vi "getSubscriberlistfromcluster.vi"(2 "add variables to subscribe":string, 3 "Data cluster out":T1) -> (0 "remote subscriber string":string, 1 "final subscriber string":string)   [LabVIEW 2013]
uses:
  dataCluster.ctl
  <vilib>/vision/Image Controls.llb/IMAQ Image.ctl
  DataQueueTypeDef.ctl
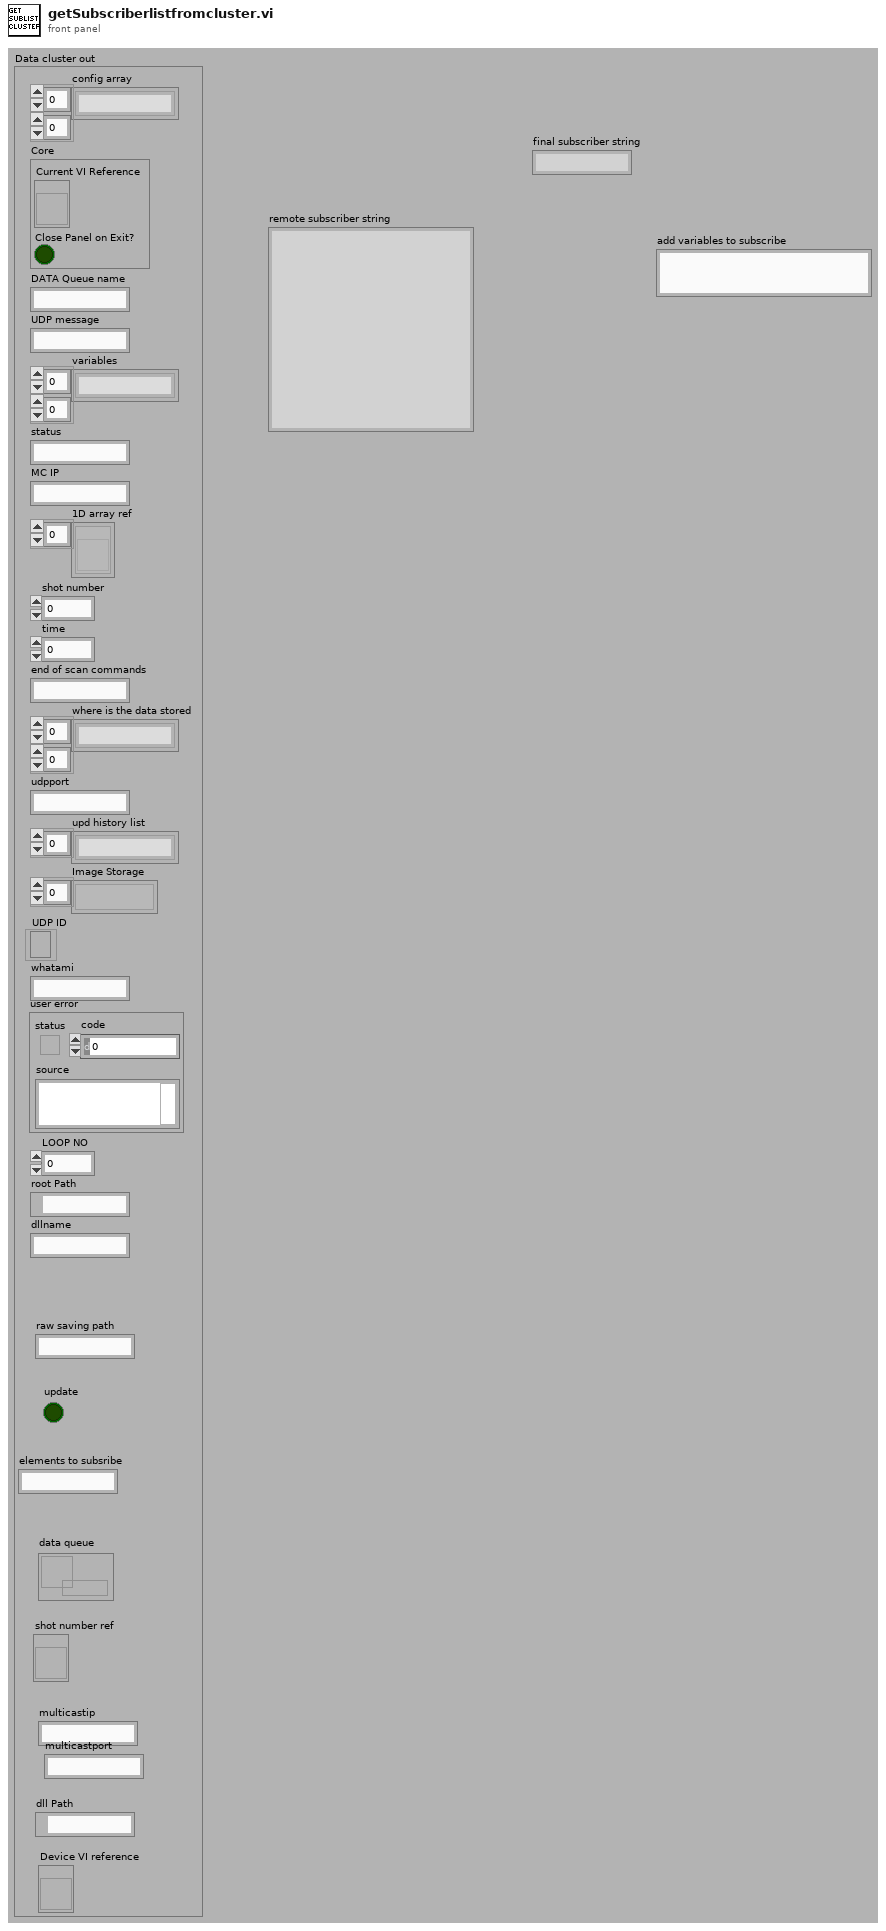
[diagram p1: front panel]
types:
  T1 = typedef "dataCluster.ctl" = cluster{"config array":string[][], "Core":cluster{"Current VI Reference":refnum<vi>, "Close Panel on Exit?":bool}, "DATA Queue name":string, "UDP message":string, "variables":string[][], "status":string, "MC IP":string, "1D array ref":refnum<vi>[], "shot number":i32, "time":u32, "end of scan commands":string, "where is the data stored":string[][], "udpport":string, "upd history list":string[], "Image Storage":T2[], "UDP ID":refnum<k16>, "whatami":string, "user error":errorcluster, "LOOP NO":u32, "root Path":path, "dllname":string, "raw saving path":string, "update":bool, "elements to subsribe":string, "data queue":refnum<queue>, "shot number ref":refnum<vi>, "multicastip":string, "multicastport":string, "dll Path":path, "Device VI reference":refnum<vi>}
  T2 = typedef "IMAQ Image.ctl" = refnum<image>
  T3 = typedef "DataQueueTypeDef.ctl" = cluster{"connection ID":refnum<k5>, "remote address":string, "Subscriber list":string[], "wait":bool, "port":u16}
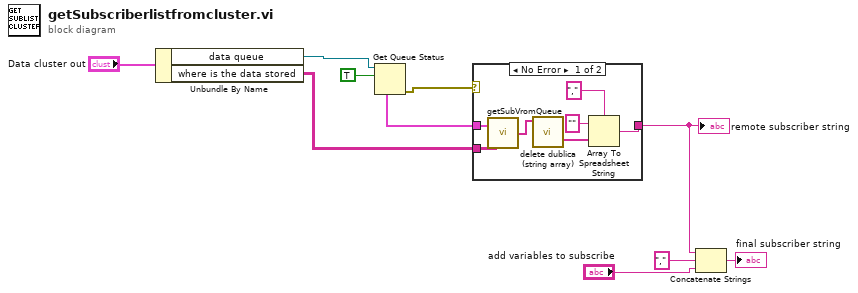
[diagram p0: block diagram]
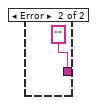
[diagram p2: hidden frame]
diagram:
  n1 = Unbundle By Name("Data cluster out") -> ("data queue"=w10:refnum<queue>, "where is the data stored"=w7:string[][])
  n2 = Get Queue Status(queue=w10, return elements? (F)=TRUE) -> (error out=w8:errorcluster, elements=w6:T3[])  [unwired: 1 in, 6 out]
  n3 = case shown="No Error" w8 {
    tunnel: w6 -> [w16 _]
    tunnel: [w12 "" ("spreadsheet string")] -> w2
    tunnel: w7 -> [w11 _]
    frame No Error {
      n4 = call "getSubVromQueue.vi"("where is the data stored"=w11, "elements"=w16) -> ("Array"=w17:string[])
      n5 = call "delete dublica (string array).vi"("Array in"=w17) -> ("Array out"=w15:string[])  [unwired: 10 in]
      n6 = Array To Spreadsheet String(delimiter (Tab)=",", array=w15, 3:"" ("format string")) -> (spreadsheet string=w12:string)
    }
    frame Error {
    }
  }
  "remote subscriber string" <- w2
  n7 = Concatenate Strings(w2, "," ("string"), "add variables to subscribe") -> (→"final subscriber string":string)
